vi "Write Setting Array.vi"(8 "error in (no error)":errorcluster, 10 "Data":u64[](array[numeric]), 11 "ScopeBase in":refnum<class "ScopeBase.lvclass">) -> (0 "error out":errorcluster, 3 "ScopeBase out":refnum<class "ScopeBase.lvclass">)   [LabVIEW 2018, in "ScopeBase.lvclass"]
uses:
  ScopeBase.lvclass
  ScopeBase.lvclass/ScopeBase.ctl
  <vilib>/Utility/error.llb/Error Cluster From Error Code.vi
  <vilib>/rvi/errors/niLvFpgaAdjustHostInterfaceError.vi
  <vilib>/rvi/interface/nirviMethod/nirviMethod.xnode
  controls/settingsFPGAref.ctl
  FpgaRef/FpgaRefBase/FpgaRefBase.lvclass
  <vilib>/FPGAPlugInAG/Dynamic/niLvFpga_WriteFifo_Dynamic.vi
  <vilib>/rvi/errors/niLvFpgaMergeErrorWithErrorCode.vi
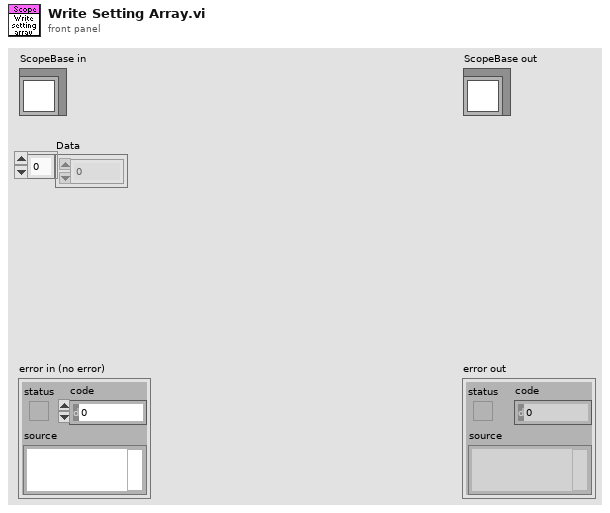
[diagram p1: front panel]
types:
  T1 = typedef "settingsFPGAref.ctl" = refnum<k20>
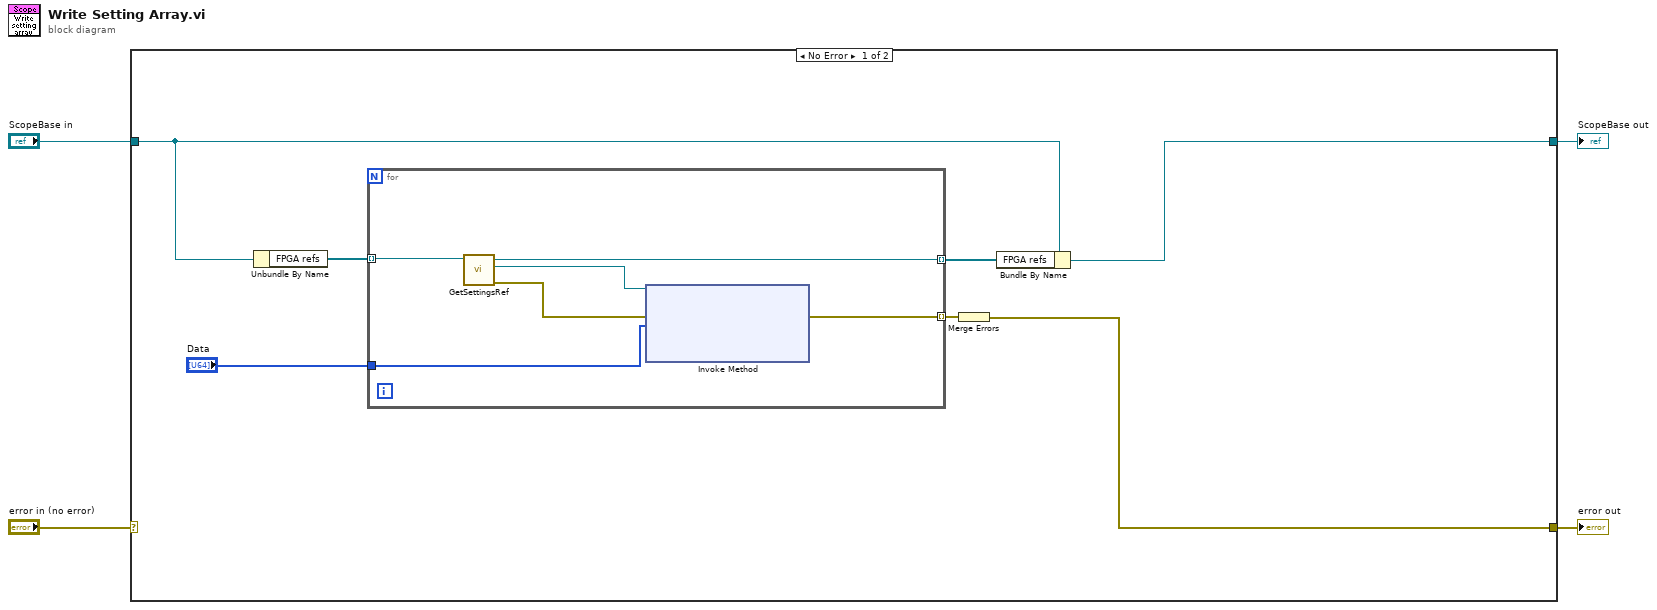
[diagram p0: block diagram]
diagram:
  n1 = case shown="No Error" "error in (no error)" {
    selector: "error in (no error)" -> [_ w18]
    tunnel: [w6 w18] -> w3
    tunnel: [w8 w17] -> w1
    tunnel: "ScopeBase in" -> [w9 w17]
    frame No Error {
      n2 = Unbundle By Name(w9) -> ("FPGA refs"=w11:refnum<class "FpgaRefBase.lvclass">[])
      n3 = for {
        tunnel: w11 -> [w16] mode=indexing
        tunnel: [w15] -> w10 mode=indexing
        tunnel: [w14] -> w7 mode=indexing
        tunnel: "Data" -> [w12]
        n4 = call-dynamic "GetSettingsRef.vi"("FpgaRefBase in"=w16) -> ("error out"=w14:errorcluster, "Settings FPGA ref"=w13:T1, "FpgaRefBase out"=w15:refnum<class "FpgaRefBase.lvclass">)  [unwired: 8 in]
        n5 = xnode "Invoke Method"("FPGA VI Reference In"=w13, "Data"=w12) -> ()  [unwired: 2 in, 3 out]
      }
      n6 = Merge Errors(w7) -> (w6:errorcluster)
      n7 = Bundle By Name(cluster=w9, "FPGA refs"=w10) -> (w8:refnum<class "ScopeBase.lvclass">)
    }
    frame Error {
    }
  }
  "error out" <- w3
  "ScopeBase out" <- w1
